vi "Resolve Address Type.vi"(8 "error in (no error)":errorcluster, 9 "Subnet Bits":i32, 10 "Address":string, 11 "Address Type":T1) -> (0 "error out":errorcluster, 2 "U32 Address":u32 format="%08x")   [LabVIEW 2020, in "Vecto.lvlib"]
uses:
  Vecto.lvlib
  Address Type.ctl
  f8bc95ce-8757-4bea-a9a5-74e77d021f7a.vi
  <vilib>/Comparison/Equal/Equal Functor/Equal Functor.lvclass
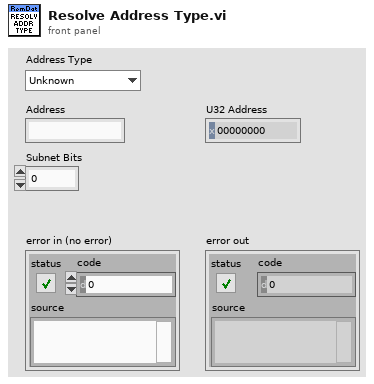
[diagram p1: front panel]
types:
  T1 = typedef "Vecto.lvlib/Address Type.ctl" = enum16{"Unknown", "Specific", "Subnet", "Any"}
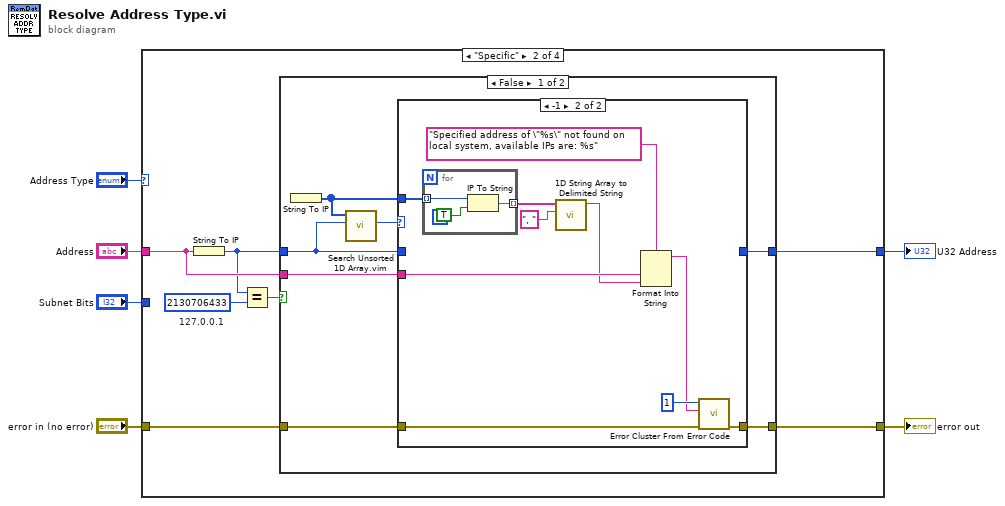
[diagram p0: block diagram]
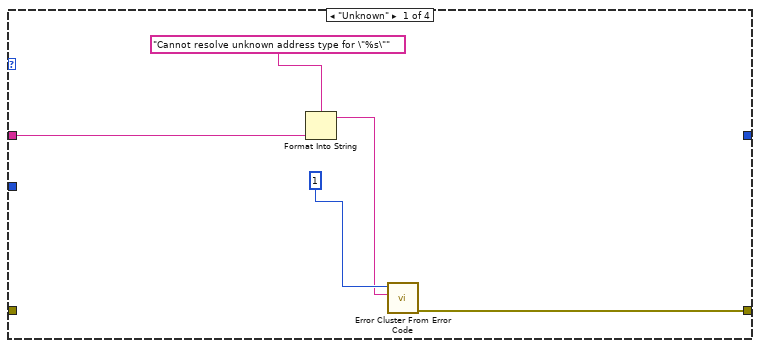
[diagram p2: hidden frame]
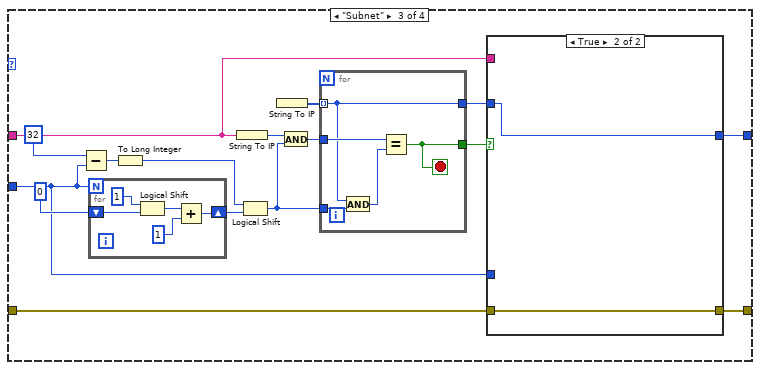
[diagram p5: hidden frame]
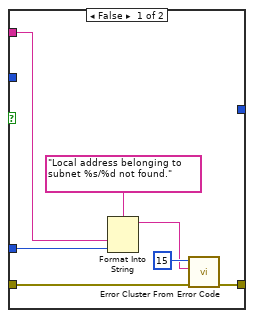
[diagram p6: hidden frame]
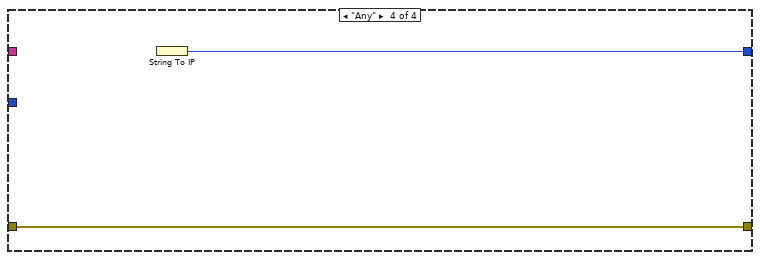
[diagram p7: hidden frame]
diagram:
  n1 = case shown="\"Specific\"" "Address Type" {
    tunnel: "Address" -> [w8 w16 w44 _]
    tunnel: "error in (no error)" -> [_ w17 w46 w78]
    tunnel: [_ w18 w47 w79] -> w3
    tunnel: [w11 w12 w45 w78] -> w2
    tunnel: "Subnet Bits" -> [_ _ w43 _]
    frame "Unknown" {
      n2 = Format Into String(format string="Cannot resolve unknown address type for \"%s\"", w8) -> (resulting string=w7:string)  [unwired: 2 in, 1 out]
      n3 = call <vilib>:"Error Cluster From Error Code.vi"("error message (\"\")"=w7, "error code (0)"=1) -> ("error out"=w11:errorcluster)  [unwired: 7 in]
    }
    frame "Specific" {
      w14 = u32 2130706433  # 127.0.0.1
      n4 = String To IP(1:w16) -> (0:w15:u32)
      n5 = Equal?(x=w15, y=w14) -> (x = y?=w13:bool)
      n6 = case shown="False" w13 {
        tunnel: [w24 w42] -> w18
        tunnel: w17 -> [w22 w41]
        tunnel: w16 -> [w20 _]
        tunnel: w15 -> [w19 w42]
        tunnel: [w23 w41] -> w12
        frame False {
          n7 = String To IP() -> (0:w21:u32[])  [unwired: 1 in]
          n8 = call "Search Unsorted 1D Array.vim"("element"=w19, "unsorted 1D array"=w21) -> ("index of element"=w25:i32)  [unwired: 9 in]
          n9 = case shown="-1" w25 {
            tunnel: w19 -> [w27 _]
            tunnel: [w27 _] -> w24
            tunnel: [w26 w33] -> w23
            tunnel: w22 -> [w26 w34]
            tunnel: w21 -> [_ w37]
            tunnel: w20 -> [_ w29]
            frame Default {
            }
            frame -1 {
              n10 = for {
                tunnel: w37 -> [w40] mode=indexing
                tunnel: [w38] -> w36 mode=indexing
                n11 = IP To String(1:TRUE ("dot notation? (F)"), 2:w40) -> (0:w38:string)
              }
              n12 = call <vilib>:"1D String Array to Delimited String.vi"("delimiter"=", ", "string array"=w36) -> ("delimited string"=w28:string)  [unwired: 9 in]
              n13 = Format Into String(format string="Specified address of \"%s\" not found on local system, available IPs are: %s", w29, w28) -> (resulting string=w31:string)  [unwired: 2 in, 1 out]
              n14 = call <vilib>:"Error Cluster From Error Code.vi"("error in (no error)"=w34, "error message (\"\")"=w31, "error code (0)"=1) -> ("error out"=w33:errorcluster)  [unwired: 6 in]
            }
          }
        }
        frame True {
        }
      }
    }
    frame "Subnet" {
      n15 = Subtract(x=32, y=w43) -> (x-y=w56:i32)
      n16 = for {
        N: w43 -> [_]
        shift-right: [w73] -> w55
        shift-left: u32 0 -> [w77]
        n17 = Logical Shift(y=i16 1, x=w77) -> (x << y=w75:u32)
        n18 = Add(x=w75, y=u32 1) -> (x+y=w73:u32)
      }
      n19 = To Long Integer(number=w56) -> (32bit integer=w54:i32)
      n20 = String To IP(1:w44) -> (0:w53:u32)
      n21 = Logical Shift(y=w54, x=w55) -> (x << y=w50:u32)
      n22 = String To IP() -> (0:w51:u32[])  [unwired: 1 in]
      n23 = And(x=w53, y=w50) -> (x .and. y?=w52:u32)
      n24 = for {
        tunnel: w52 -> [w71]
        tunnel: w51 -> [w69] mode=indexing
        tunnel: w50 -> [w72]
        tunnel: [w69] -> w49
        tunnel: [w68] -> w48
        stop <- w68 stop-if-true
        n25 = And(x=w69, y=w72) -> (x .and. y?=w70:u32)
        n26 = Equal?(x=w71, y=w70) -> (x = y?=w68:bool)
      }
      n27 = case shown="True" w48 {
        tunnel: w49 -> [_ w67]
        tunnel: [_ w67] -> w47
        tunnel: w46 -> [w65 w66]
        tunnel: [w64 w66] -> w45
        tunnel: w44 -> [w61 _]
        tunnel: w43 -> [w62 _]
        frame False {
          n28 = Format Into String(format string="Local address belonging to subnet %s/%d not found.", w61, w62) -> (resulting string=w59:string)  [unwired: 2 in, 1 out]
          n29 = call <vilib>:"Error Cluster From Error Code.vi"("error in (no error)"=w65, "error message (\"\")"=w59, "error code (0)"=15) -> ("error out"=w64:errorcluster)  [unwired: 6 in]
        }
        frame True {
        }
      }
    }
    frame "Any" {
      n30 = String To IP() -> (0:w79:u32)  [unwired: 1 in]
    }
  }
  "error out" <- w2
  "U32 Address" <- w3
